vi "TANKI_PID_ARDUINO.vi"() -> ()   [LabVIEW 2021]
uses:
  <vilib>/Instr/_visa.llb/VISA Configure Serial Port (Instr).vi
panel:
  out "Loop":i32
  in  "Auto SetPoint":bool
  out "millisecond timer value":u32
  in  "COM Port":refnum<visa-resource-name>
  in  "File Path":path
  out "KD_":dbl
  out "KI_":dbl
  out "KP_":dbl
  out "Level":dbl
  out "Error":dbl
  in  "Valve (liter/detik)":u16(slide) scale=0.0..5.0
  in  "Disturbance (Liter/Detik)":dbl(knob) min=0.0 max=10.0 step=1.0 scale=0.0..10.0
  out "Grafik sistem":dynamicdata(graph)
  in  "Stop Button":bool
  in  "KD":dbl(knob) min=0.0 max=100.0 step=0.1 scale=0.0..1.0
  in  "KI":dbl(knob) min=0.0 max=100.0 step=0.1 scale=0.0..1.0
  in  "KP":dbl(knob) min=0.0 max=100.0 step=0.1 scale=0.0..1.0
  out "Level Tanki":dbl
  out "Pompa (Liter/Detik)":dbl(knob) scale=0.0..30.0
  in  "Set Point":u16(slide) max=500 step=1 scale=0.0..500.0
  out "Tank":dbl(slide) scale=0.0..500.0
  # "D4 TEKNOLOGI REKAYASA INSTRUMENTASI DAN KONTROL SV UGM"
  # "SIMULASI HIL KENDALI LEVEL TANKI"
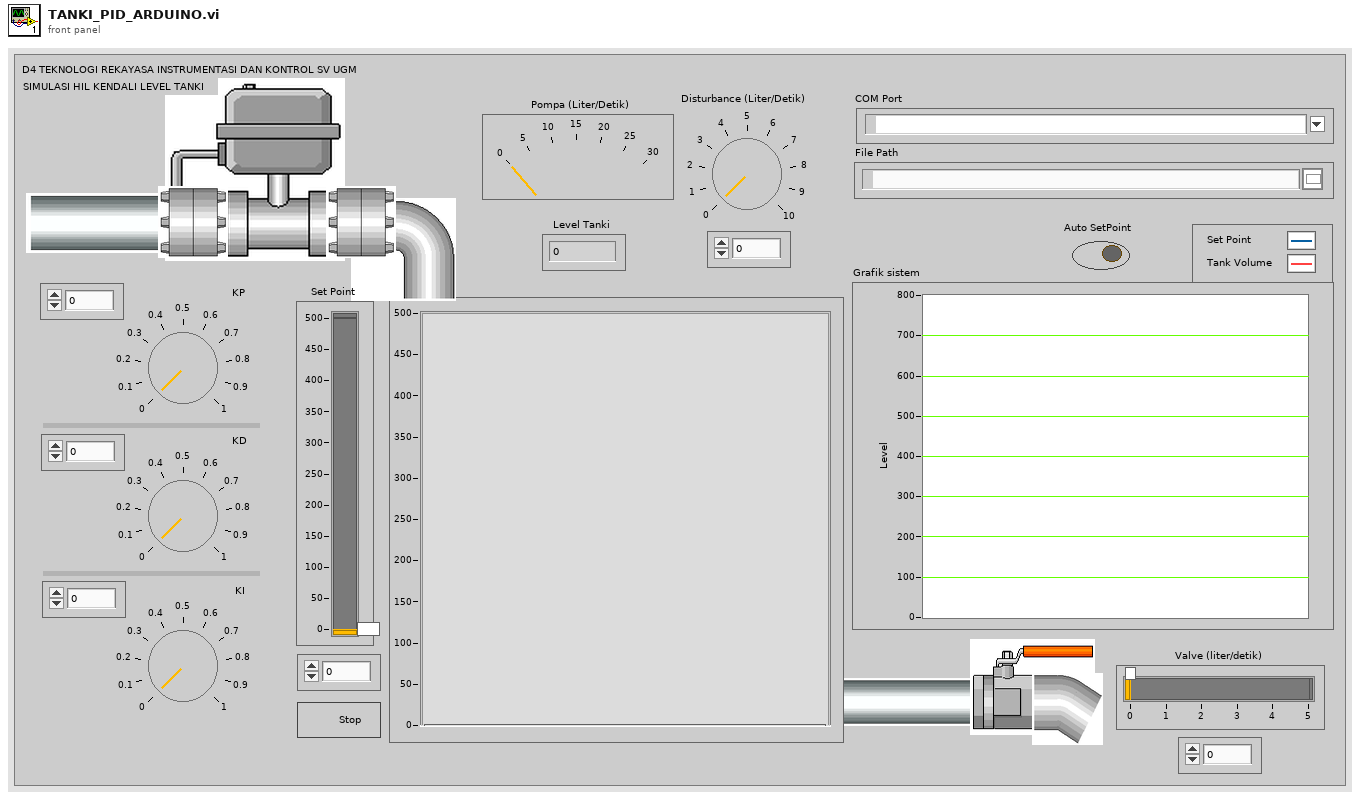
[diagram p1: front panel]
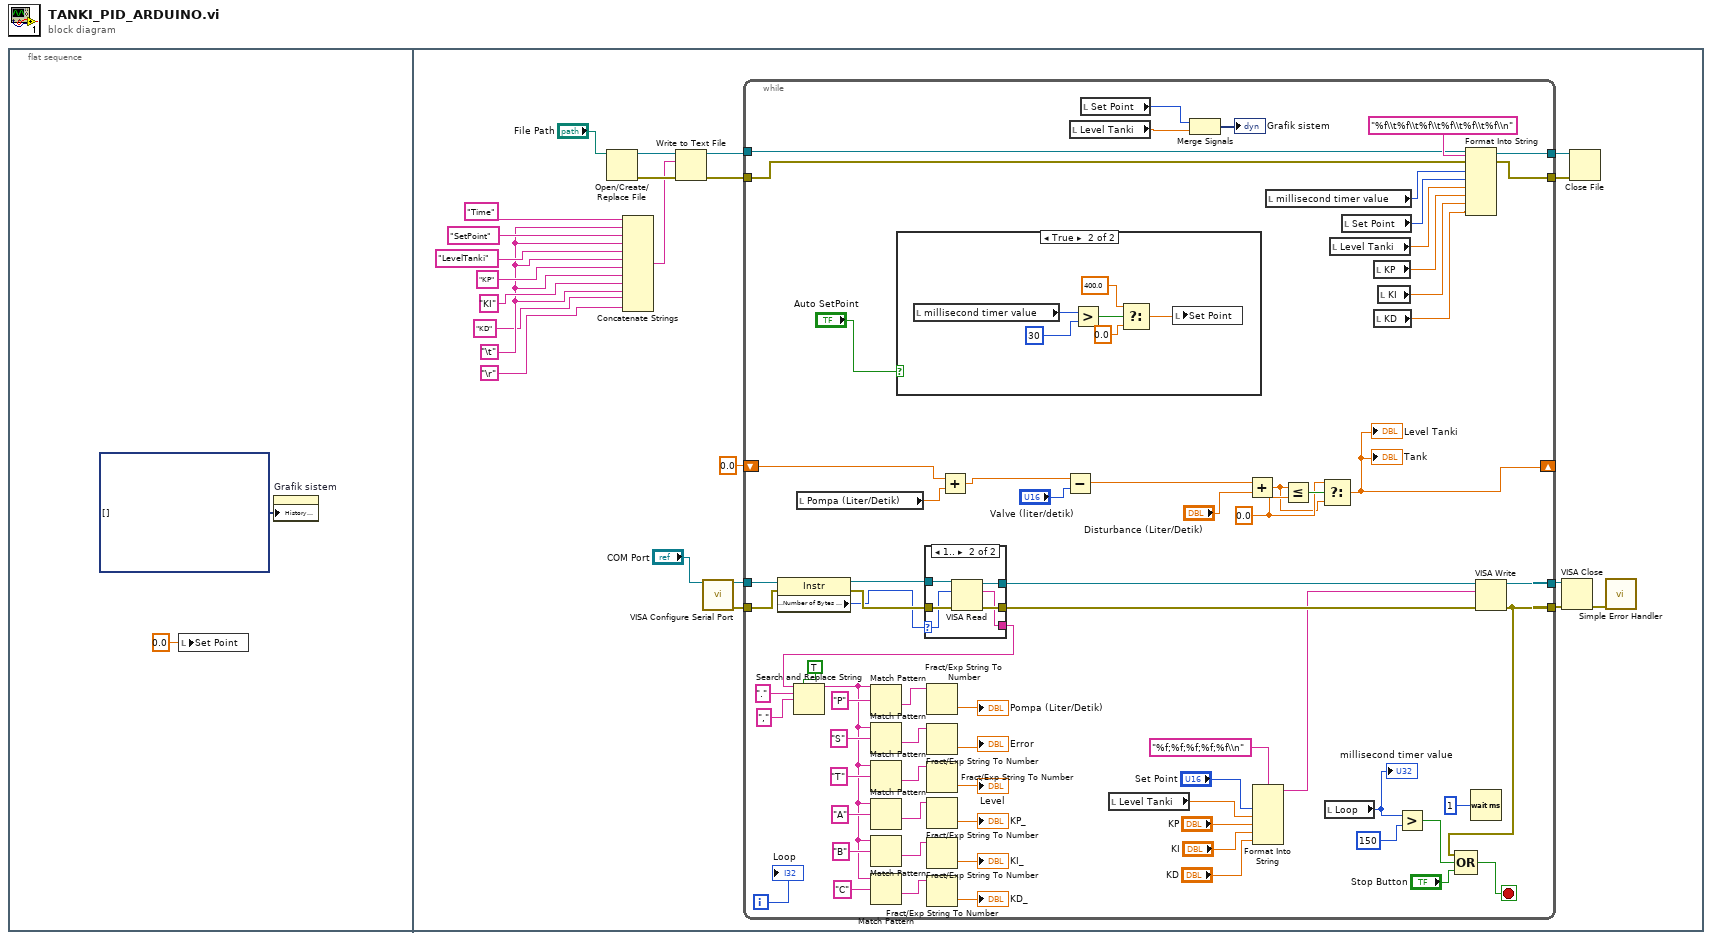
[diagram p0: block diagram]
diagram:
  n1 = flat-sequence {
    frame #0 {
      n2 = local write "Set Point"(0.0 ("Set Point")) -> ()
      n3 = property on="Grafik sistem" class="WFChart (strict)"("History Data"=dynamicdata[] []) -> ()  [unwired: 2 in, 2 out]
    }
    frame #1 {
      w5 = "\t"
      n4 = Open/Create/Replace File(file path (use dialog)="File Path") -> (refnum out=w15:refnum<file>, error out=w14:errorcluster)  [unwired: 5 in, 1 out]
      n5 = Concatenate Strings("Time" ("text"), w5, "SetPoint" ("text"), w5, "LevelTanki" ("string"), w5, "KP" ("string"), w5, "KI" ("string"), w5, "KD" ("string"), "\r") -> (w10:string)
      n6 = Write to Text File(file (use dialog)=w15, text=w10, error in=w14) -> (refnum out=w12:refnum<file>, error out=w13:errorcluster)  [unwired: 1 in, 1 out]
      n7 = call-poly "VISA Configure Serial Port"("VISA resource name"="COM Port") -> ("VISA resource name out"=w24:refnum<visa-resource-name>, "error out"=w23:errorcluster)  [unwired: 13 in]
      n8 = while {
        shift-right: [w87] -> _
        shift-left: 0.0 ("t") -> [w96]
        tunnel: w24 -> [w84]
        tunnel: w23 -> [w83]
        tunnel: [w79] -> w22
        tunnel: [w68] -> w21
        tunnel: [w41] -> w19
        tunnel: [w40] -> w18
        tunnel: w12 -> [w39]
        tunnel: w13 -> [w38]
        i -> [w30]
        stop <- w73 stop-if-true
        w86 = 0.0 ("y")
        n9 = property class="Instr"(reference=w84, error in=w83) -> (reference out=w82:refnum<visa-resource-name>, error out=w81:errorcluster, "Serial Settings:Number of Bytes at Serial Port"=w78:u32)
        n10 = local read "Pompa (Liter/Detik)"() -> (w52:dbl)
        n11 = case shown="True" "Auto SetPoint" {
          frame False {
          }
          frame True {
            n12 = local read "millisecond timer value"() -> (w102:u32)
            n13 = Greater?(x=w102, y=u32 30) -> (0:w100:bool)
            n14 = Select(t=400.0, s=w100, f=0.0) -> (s? t:f=w97:dbl)
            n15 = local write "Set Point"(w97) -> ()
          }
        }
        n16 = case shown="1.." w78 {
          selector: w78 -> [_ w105]
          tunnel: w82 -> [w104 w110]
          tunnel: w81 -> [w103 w109]
          tunnel: [w104 w108] -> w80
          tunnel: [w103 w107] -> w74
          tunnel: [_ w106] -> w67
          frame 0, Default {
          }
          frame 1.. {
            n17 = VISA Read(VISA resource name=w110, byte count=w105, error in (no error)=w109) -> (VISA resource name out=w108:refnum<visa-resource-name>, read buffer=w106:string, error out=w107:errorcluster)  [unwired: 1 out]
          }
        }
        n18 = Search and Replace String(replace all?=TRUE ("replace all? (F)"), input string=w67, search string=".", replace string="," ("replace string (\"\")")) -> (result string=w60:string)  [unwired: 4 in, 3 out]
        n19 = Match Pattern(string=w60, regular expression="P") -> (after substring=w59:string)  [unwired: 1 in, 3 out]
        n20 = Match Pattern(string=w60, regular expression="S") -> (after substring=w58:string)  [unwired: 1 in, 3 out]
        n21 = Match Pattern(string=w60, regular expression="T") -> (after substring=w57:string)  [unwired: 1 in, 3 out]
        n22 = Match Pattern(string=w60, regular expression="A") -> (after substring=w56:string)  [unwired: 1 in, 3 out]
        n23 = Match Pattern(string=w60, regular expression="B") -> (after substring=w55:string)  [unwired: 1 in, 3 out]
        n24 = Match Pattern(string=w60, regular expression="C") -> (after substring=w54:string)  [unwired: 1 in, 3 out]
        n25 = Fract/Exp String To Number(string=w59) -> (number=→"Pompa (Liter/Detik)":dbl)  [unwired: 3 in, 1 out]
        n26 = Fract/Exp String To Number(string=w58) -> (number=→"Error":dbl)  [unwired: 3 in, 1 out]
        n27 = Fract/Exp String To Number(string=w57) -> (number=→"Level":dbl)  [unwired: 3 in, 1 out]
        n28 = Fract/Exp String To Number(string=w56) -> (number=→"KP_":dbl)  [unwired: 3 in, 1 out]
        n29 = Fract/Exp String To Number(string=w55) -> (number=→"KI_":dbl)  [unwired: 3 in, 1 out]
        n30 = Fract/Exp String To Number(string=w54) -> (number=→"KD_":dbl)  [unwired: 3 in, 1 out]
        n31 = Add(x=w96, y=w52) -> (x+y=w95:dbl)
        n32 = Subtract(x=w95, y="Valve (liter/detik)") -> (x-y=w90:dbl)
        n33 = local read "Level Tanki"() -> (w92:dbl)
        n34 = local read "Set Point"() -> (w93:u16)
        n35 = local read "Level Tanki"() -> (w51:dbl)
        n36 = Merge Signals(w93, w92) -> (→"Grafik sistem":dynamicdata)
        n37 = Add(x=w90, y="Disturbance (Liter/Detik)") -> (x+y=w85:dbl)
        n38 = Format Into String(format string="%f;%f;%f;%f;%f\\n", "Set Point", w51, "KP", "KI", "KD") -> (resulting string=w69:string)  [unwired: 2 in, 1 out]
        n39 = local read "millisecond timer value"() -> (w32:u32)
        n40 = Less Or Equal?(x=w85, y=w86) -> (x <= y?=w88:bool)
        n41 = Select(t=w86, s=w88, f=w85) -> (s? t:f=w87:dbl)
        "Tank" <- w87
        "Level Tanki" <- w87
        n42 = local read "Loop"() -> (w29:i32)
        "millisecond timer value" <- w29
        n43 = local read "Level Tanki"() -> (w36:dbl)
        n44 = local read "Set Point"() -> (w37:u16)
        n45 = local read "KP"() -> (w28:dbl)
        n46 = local read "KD"() -> (w26:dbl)
        n47 = local read "KI"() -> (w27:dbl)
        n48 = Greater?(x=w29, y=u32 150 ("x")) -> (0:w33:bool)
        n49 = Format Into String(format string="%f\\t%f\\t%f\\t%f\\t%f\\t%f\\n", initial string=w39, error in=w38, w32, w37, w36, w28, w27, w26) -> (resulting string=w41:refnum<file>, error out=w40:errorcluster)
        n50 = Wait (ms)(milliseconds to wait=u32 1) -> ()  [unwired: 1 out]
        n51 = VISA Write(VISA resource name=w80, write buffer=w69, error in (no error)=w74) -> (VISA resource name out=w79:refnum<visa-resource-name>, error out=w68:errorcluster)  [unwired: 1 out]
        n52 = Compound Arithmetic op=OR(w68, w33, "Stop Button") -> (w73:bool)
        "Loop" <- w30
      }
      n53 = VISA Close(VISA resource name=w22, error in (no error)=w21) -> (error out=w20:errorcluster)
      n54 = Close File(refnum=w19, error in=w18) -> ()  [unwired: 2 out]
      n55 = call <vilib>:"Simple Error Handler.vi"("error in (no error)"=w20) -> ()  [unwired: 4 in, 5 out]
    }
  }
